vi "Lookup Message Channels.vi"(8 "error in (no error)":errorcluster, 10 "Message Channels in":T3 {"Status" format="%.0x"; "Triggers" format="%.0x"; "Periodic Enable" format="%.0x"}, 11 "Section Ref in":T2 format="%.0x") -> (0 "error out":errorcluster, 1 "Trigger Parameters":T1, 2 "Message Channels out":T3 {"Status" format="%.0x"; "Triggers" format="%.0x"; "Periodic Enable" format="%.0x"}, 3 "Section Ref out":T2 format="%.0x")   [LabVIEW 2018, in "Instrument Addon System Explorer.lvlib"]
uses:
  Instrument Addon System Explorer.lvlib
  <vilib>/NI VeriStand/Custom Device Tools/Custom Device Utility Library/Custom Device Utility Library.lvlib
  <vilib>/NI VeriStand/Custom Device Tools/Custom Device Utility Library/NI VeriStand - Search for Item by GUID.vi
  Addon Shared/SubVIs/Constants.vi
  Addon Shared/Instrument Addon Shared.lvlib
  Addon Shared/Types/FG Control.ctl
  <vilib>/NI VeriStand/Custom Device API/Custom Device Item Ref.ctl
  <vilib>/NI VeriStand/Custom Device API/Custom Device API.lvlib
  Types/Message Channel Lookup Cluster.ctl
  Addon Shared/Types/Trigger Parameters.ctl
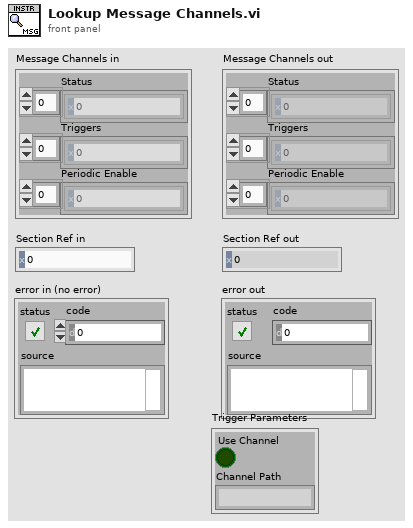
[diagram p1: front panel]
types:
  T1 = typedef "Instrument Addon Shared.lvlib/Trigger Parameters.ctl" = cluster{"Use Channel":bool, "Channel Path":string}
  T2 = typedef "Custom Device API.lvlib/Custom Device Item Ref.ctl" = u64
  T3 = typedef "Instrument Addon System Explorer.lvlib/Message Channel Lookup Cluster.ctl" = cluster{"Status":T2[], "Triggers":T2[], "Periodic Enable":T2[]}
  T4 = typedef "Instrument Addon Shared.lvlib/FG Control.ctl" = enum16{"Get", "Set"}
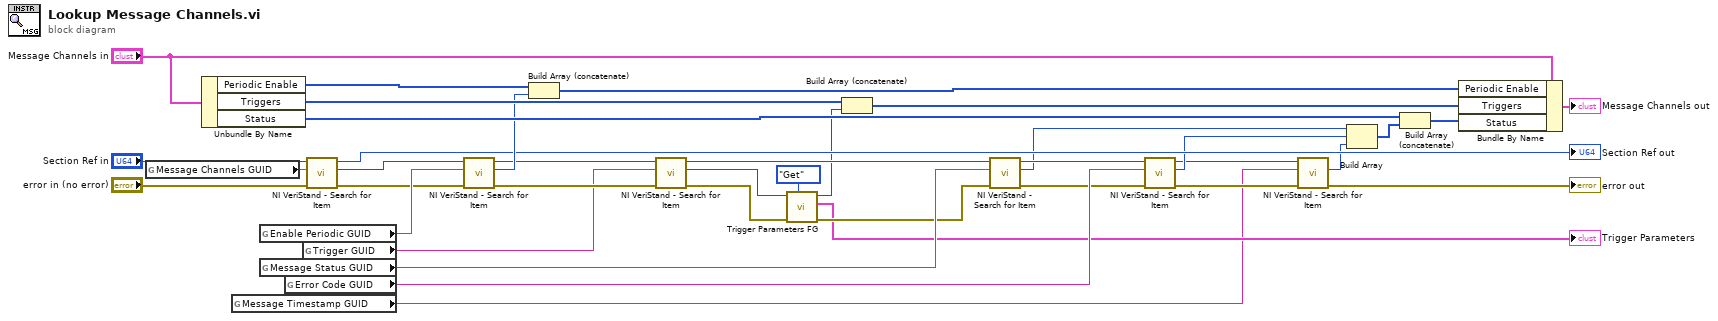
[diagram p0: block diagram]
diagram:
  n1 = global read "Constants.vi" "Message Channels GUID"() -> (w14:string)
  n2 = Unbundle By Name("Message Channels in") -> ("Periodic Enable"=w33:T2[], "Triggers"=w34:T2[], "Status"=w35:T2[])
  n3 = global read "Constants.vi" "Message Timestamp GUID"() -> (w2:string)
  n4 = global read "Constants.vi" "Enable Periodic GUID"() -> (w31:string)
  n5 = global read "Constants.vi" "Message Status GUID"() -> (w19:string)
  n6 = global read "Constants.vi" "Error Code GUID"() -> (w18:string)
  n7 = global read "Constants.vi" "Trigger GUID"() -> (w20:string)
  n8 = call-poly <vilib>:"NI VeriStand - Search for Item.vi"("error in"="error in (no error)", "Item GUID"=w14, "Section Ref in"="Section Ref in") -> ("error out"=w29:errorcluster, "Item Ref"=w27:T2, "Section Ref out"=→"Section Ref out":T2)  [unwired: 5 in, 1 out]
  n9 = call-poly <vilib>:"NI VeriStand - Search for Item.vi"("error in"=w29, "Item GUID"=w31, "Section Ref in"=w27) -> ("error out"=w30:errorcluster, "Item Ref"=w32:T2, "Section Ref out"=w28:T2)  [unwired: 5 in, 1 out]
  n10 = Build Array (concatenate)(w33, w32) -> (w36:T2[])
  n11 = call-poly <vilib>:"NI VeriStand - Search for Item.vi"("error in"=w30, "Item GUID"=w20, "Section Ref in"=w28) -> ("error out"=w8:errorcluster, "Item Ref"=w11:T2, "Section Ref out"=w17:T2)  [unwired: 5 in, 1 out]
  n12 = call "Trigger Parameters FG.vi"("Action"=FG_Control."Get", "error in (no error)"=w8, "Item Ref in"=w11) -> ("error out"=w7:errorcluster, "Trigger Parameters"=→"Trigger Parameters":T1, "Item Ref out"=w10:T2)  [unwired: 6 in]
  n13 = Build Array (concatenate)(w34, w10) -> (w12:T2[])
  n14 = call-poly <vilib>:"NI VeriStand - Search for Item.vi"("error in"=w7, "Item GUID"=w19, "Section Ref in"=w17) -> ("error out"=w16:errorcluster, "Item Ref"=w21:T2, "Section Ref out"=w26:T2)  [unwired: 5 in, 1 out]
  n15 = call-poly <vilib>:"NI VeriStand - Search for Item.vi"("error in"=w16, "Item GUID"=w18, "Section Ref in"=w26) -> ("error out"=w4:errorcluster, "Item Ref"=w22:T2, "Section Ref out"=w5:T2)  [unwired: 5 in, 1 out]
  n16 = call-poly <vilib>:"NI VeriStand - Search for Item.vi"("error in"=w4, "Item GUID"=w2, "Section Ref in"=w5) -> ("error out"=→"error out":errorcluster, "Item Ref"=w1:T2)  [unwired: 5 in, 2 out]
  n17 = Build Array(w21, w22, w1) -> (w23:T2[])
  n18 = Build Array (concatenate)(w35, w23) -> (w13:T2[])
  n19 = Bundle By Name(cluster="Message Channels in", "Periodic Enable"=w36, "Triggers"=w12, "Status"=w13) -> (→"Message Channels out":T3)
